vi "Lockin.DAQ.Generate.Waveforms.vi"(4 "sweep index":i32=-1, 6 "Reset?":bool, 8 "error in (no error)":errorcluster, 11 "Lockin.DAQ":refnum<class "Lockin.DAQ.lvclass">) -> (0 "error out":errorcluster, 1 "REF []":waveform(dbl)[](array[waveform]), 2 "AO []":waveform(dbl)[](array[waveform]), 3 "Lockin.DAQ":refnum<class "Lockin.DAQ.lvclass">, 5 "Sweep []":waveform(dbl)[](array[waveform]))   [LabVIEW 2016, in "Lockin.DAQ.lvclass"]
uses:
  Lockin.DAQ.lvclass
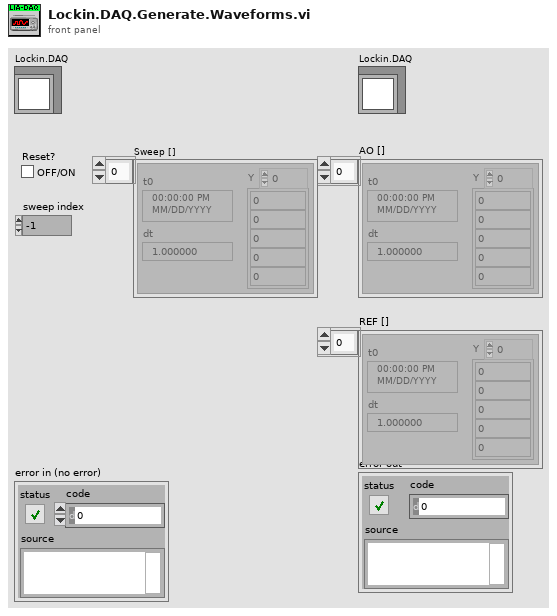
[diagram p1: front panel]
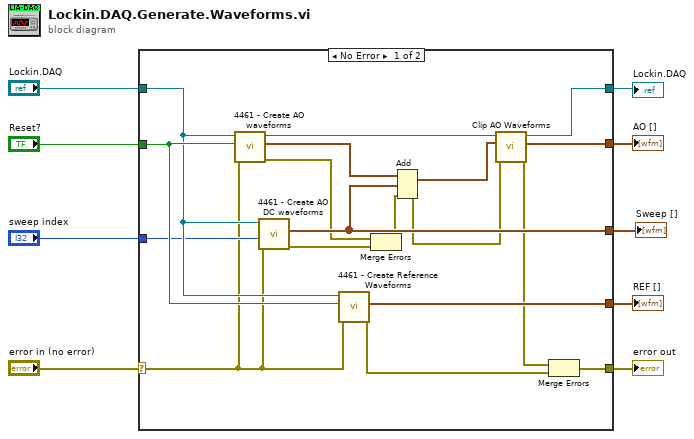
[diagram p0: block diagram]
diagram:
  n1 = case shown="No Error" "error in (no error)" {
    selector: "error in (no error)" -> [w16 w29]
    tunnel: [w27 _] -> w9
    tunnel: "Reset?" -> [w26 _]
    tunnel: [w25 _] -> w7
    tunnel: [w24 w29] -> w6
    tunnel: "Lockin.DAQ" -> [w23 w28]
    tunnel: "sweep index" -> [w21 _]
    tunnel: [w17 _] -> w3
    tunnel: [w18 w28] -> w2
    frame No Error {
      n2 = call "4461 - Create AO waveforms.vi"("error in (no error)"=w16, "reset signal"=w26, "Lockin.DAQ"=w23) -> ("error out"=w11:errorcluster, "AO Array"=w20:waveform(dbl)[], "Lockin.DAQ"=w19:refnum<class "Lockin.DAQ.lvclass">)  [unwired: 5 in, 1 out]
      n3 = call "4461 - Create AO DC waveforms.vi"("error in (no error)"=w16, "sweep index"=w21, "Lockin.DAQ in"=w23) -> ("error out"=w13:errorcluster, "AO Array"=w17:waveform(dbl)[])  [unwired: 6 in, 1 out]
      n4 = call "4461 - Create Reference Waveforms.vi"("error in (no error)"=w16, "reset signal"=w26, "LockinDAQ"=w23) -> ("error out"=w15:errorcluster, "Ref Array"=w27:waveform(dbl)[])  [unwired: 5 in, 2 out]
      n5 = Merge Errors(w11, w13) -> (w12:errorcluster)
      n6 = Add(1:w17, 2:w20, 4:w12) -> (0:w22:waveform(dbl)[], 3:w10:errorcluster)
      n7 = call "Clip AO Waveforms.vi"("error in (no error)"=w10, "AO []"=w22, "Lockin.DAQ in"=w19) -> ("error out"=w14:errorcluster, "Clipped AO []"=w25:waveform(dbl)[], "Lockin.DAQ out"=w18:refnum<class "Lockin.DAQ.lvclass">)  [unwired: 6 in]
      n8 = Merge Errors(w14, w15) -> (w24:errorcluster)
    }
    frame Error {
    }
  }
  "error out" <- w6
  "REF []" <- w9
  "AO []" <- w7
  "Lockin.DAQ" <- w2
  "Sweep []" <- w3
